vi "getFPGAReference.vi"(11 "Modbus in":refnum<class "Modbus.lvclass">) -> (2 "FPGAReference":refnum<k20>, 3 "Modbus out":refnum<class "Modbus.lvclass">)   [LabVIEW 2015]
uses:
  Modbus.lvclass
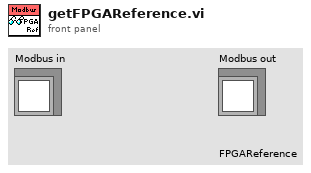
[diagram p1: front panel]
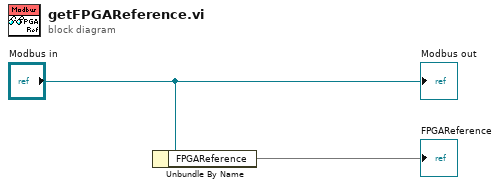
[diagram p0: block diagram]
diagram:
  n1 = Unbundle By Name("Modbus in") -> ("FPGAReference"=→"FPGAReference")
  "Modbus out" <- "Modbus in"
